vi "Init SPI.vi"(5 "Data Bits":i8=8, 7 "Mode":T1, 8 "error in (no error)":errorcluster, 9 "Baud":u32=1000000 format="%.0p", 10 "SPI #":T2=-1, 11 "Session in":refnum<class "Session.lvclass">) -> (0 "error out":errorcluster, 3 "Session out":refnum<class "Session.lvclass">)   [LabVIEW 2024, in "CTI.lvlib" / "Session.lvclass"]
uses:
  Session.lvclass
  SPI Number.ctl
  SPI Mode.ctl
  SPI Config.ctl
  SPI Pins.ctl
  GPIO Number.ctl
  DeviceComms/DeviceComms.lvclass
  CTI.lvlib
  SPI/SPI.lvclass
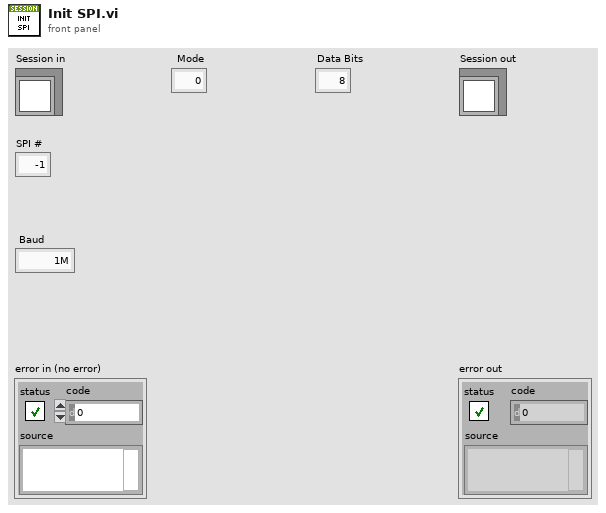
[diagram p1: front panel]
types:
  T1 = typedef "CTI.lvlib/SPI Mode.ctl" = i8
  T2 = typedef "CTI.lvlib/SPI Number.ctl" = i8
  T3 = typedef "CTI.lvlib/GPIO Number.ctl" = i8
  T4 = typedef "CTI.lvlib/SPI Config.ctl" = cluster{"Mode":T1, "Data Bits":i8, "Pins":T5}
  T5 = typedef "CTI.lvlib/SPI Pins.ctl" = cluster{"TX GPIO":T3, "RX GPIO":T3, "SCK GPIO":T3}
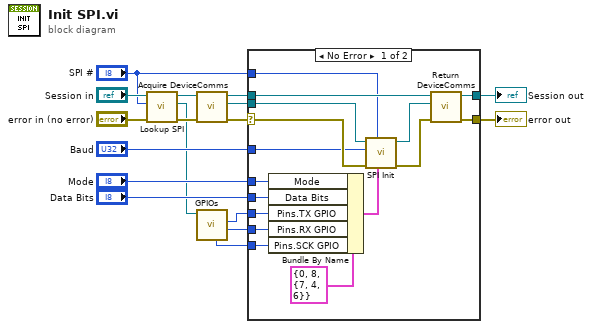
[diagram p0: block diagram]
diagram:
  n1 = call "Lookup SPI.vi"("error in (no error)"="error in (no error)", "SPI #"="SPI #", "Session in"="Session in") -> ("error out"=w5:errorcluster, "SPI"=w2:refnum<class "SPI.lvclass">, "Session out"=w3:refnum<class "Session.lvclass">)  [unwired: 6 in]
  n2 = call "Acquire DeviceComms.vi"("error in (no error)"=w5, "Session in"=w3) -> ("error out"=w17:errorcluster, "DeviceComms"=w12:refnum<class "DeviceComms.lvclass">, "Session out"=w10:refnum<class "Session.lvclass">)  [unwired: 7 in]
  n3 = call "GPIOs.vi"("SPI in"=w2) -> ("RX GPIO"=w7:T3, "TX GPIO"=w8:T3, "SCK GPIO"=w6:T3)  [unwired: 6 in, 2 out]
  n4 = case shown="No Error" w17 {
    selector: w17 -> [w33 w34]
    tunnel: "Mode" -> [w30 _]
    tunnel: "Data Bits" -> [w29 _]
    tunnel: "Baud" -> [w28 _]
    tunnel: w12 -> [w27 _]
    tunnel: [w26 w34] -> w11
    tunnel: w10 -> [w25 w35]
    tunnel: [w24 w35] -> w9
    tunnel: "SPI #" -> [w21 _]
    tunnel: w8 -> [w20 _]
    tunnel: w7 -> [w19 _]
    tunnel: w6 -> [w18 _]
    frame No Error {
      n5 = Bundle By Name(cluster=T4 {"Mode"=0, "Data Bits"=8, "Pins"={"TX GPIO"=7, "RX GPIO"=4, "SCK GPIO"=6}} ("SPI Config"), "Mode"=w30, "Data Bits"=w29, "Pins.TX GPIO"=w20, "Pins.RX GPIO"=w19, "Pins.SCK GPIO"=w18) -> (w31:T4)
      n6 = call-dynamic "SPI Init.vi"("SPI Config"=w31, "SPI #"=w21, "error in (no error)"=w33, "Baud"=w28, "DeviceComms in"=w27) -> ("error out"=w23:errorcluster, "DeviceComms out"=w22:refnum<class "DeviceComms.lvclass">)  [unwired: 5 in]
      n7 = call "Return DeviceComms.vi"("error in (no error)"=w23, "DeviceComms"=w22, "Session in"=w25) -> ("error out"=w26:errorcluster, "Session out"=w24:refnum<class "Session.lvclass">)  [unwired: 7 in]
    }
    frame Error {
    }
  }
  "error out" <- w11
  "Session out" <- w9
